vi "SIFT.vi"() -> ()   [LabVIEW 2018]
doc: "SIFT: This example is the SIFT feature detection example, which reads the image and converts it into a grayscale image, instantiates SIFT, detects key points, and draws the key point detection results on the image (only the middle point is drawn for each key point)"
uses:
  vi.lib/VIRobotics/opencv_yiku/ctls/KeyPoint.ctl
  vi.lib/VIRobotics/opencv_yiku/ctls/Point2f.ctl
  vi.lib/VIRobotics/opencv_yiku/ctls/ColorConversionCodes.ctl
  vi.lib/VIRobotics/opencv_yiku/Mat/Mat_8U/Mat_8U.lvclass
  C:/Program Files/National Instruments/LabVIEW 2018/vi.lib/VIRobotics/opencv_yiku/Mat/Mat/Mat.lvclass
  vi.lib/VIRobotics/opencv_yiku/Mat/Create_Mat_8U.vi
  vi.lib/VIRobotics/opencv_yiku/features2d/vector_KeyPoints/vector_KeyPoint_get_KeyPoints.vi
  vi.lib/VIRobotics/opencv_yiku/opencv_yiku.lvlib
  vi.lib/VIRobotics/opencv_yiku/features2d/SIFT/SIFT.lvclass
  vi.lib/VIRobotics/opencv_yiku/features2d/vector_KeyPoints/vector_KeyPoint.lvclass
panel:
  in  "nfeatures":i32=100
  out "src":picture
  out "SIFT_pic":picture
  out "KeyPoints1":T1[](array[typedef])
  # "Overview: Demonstrates how to find SIFT Keypoints and Descriptors\nRequirements: Windows.\nInstructions: \n1.Run the VI"
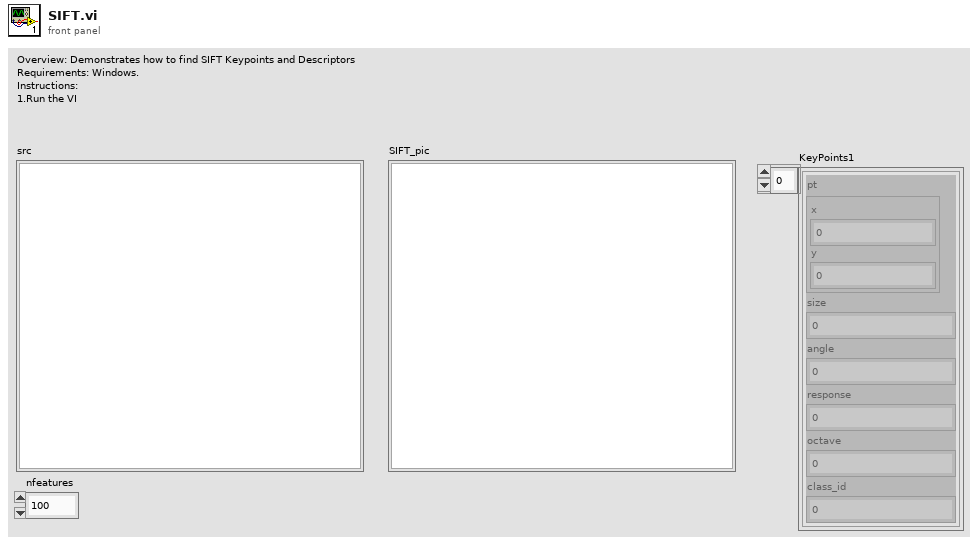
[diagram p1: front panel]
types:
  T1 = typedef "opencv_yiku.lvlib/KeyPoint.ctl" = cluster{"pt":T2, "size":sgl, "angle":sgl, "response":sgl, "octave":i32, "class_id":i32}
  T2 = typedef "opencv_yiku.lvlib/Point2f.ctl" = cluster{"x":sgl, "y":sgl}
  T3 = typedef "opencv_yiku.lvlib/ColorConversionCodes.ctl" = enum32{"COLOR_BGR2BGRA", "COLOR_BGRA2BGR", "COLOR_BGR2RGBA", "COLOR_RGBA2BGR", "COLOR_BGR2RGB", "COLOR_BGRA2RGBA", "COLOR_BGR2GRAY", "COLOR_RGB2GRAY", "COLOR_GRAY2BGR", "COLOR_GRAY2BGRA", "COLOR_BGRA2GRAY", "COLOR_RGBA2GRAY", "COLOR_BGR2BGR565", "COLOR_RGB2BGR565", "COLOR_BGR5652BGR", "COLOR_BGR5652RGB", "COLOR_BGRA2BGR565", "COLOR_RGBA2BGR565", "COLOR_BGR5652BGRA", "COLOR_BGR5652RGBA", "COLOR_GRAY2BGR565", "COLOR_BGR5652GRAY", "COLOR_BGR2BGR555", "COLOR_RGB2BGR555", "COLOR_BGR5552BGR", "COLOR_BGR5552RGB", "COLOR_BGRA2BGR555", "COLOR_RGBA2BGR555", "COLOR_BGR5552BGRA", "COLOR_BGR5552RGBA", "COLOR_GRAY2BGR555", "COLOR_BGR5552GRAY", "COLOR_BGR2XYZ", "COLOR_RGB2XYZ", "COLOR_XYZ2BGR", "COLOR_XYZ2RGB", "COLOR_BGR2YCrCb", "COLOR_RGB2YCrCb", "COLOR_YCrCb2BGR", "COLOR_YCrCb2RGB", "COLOR_BGR2HSV", "COLOR_RGB2HSV", "42", "43", "COLOR_BGR2Lab", "COLOR_RGB2Lab"}
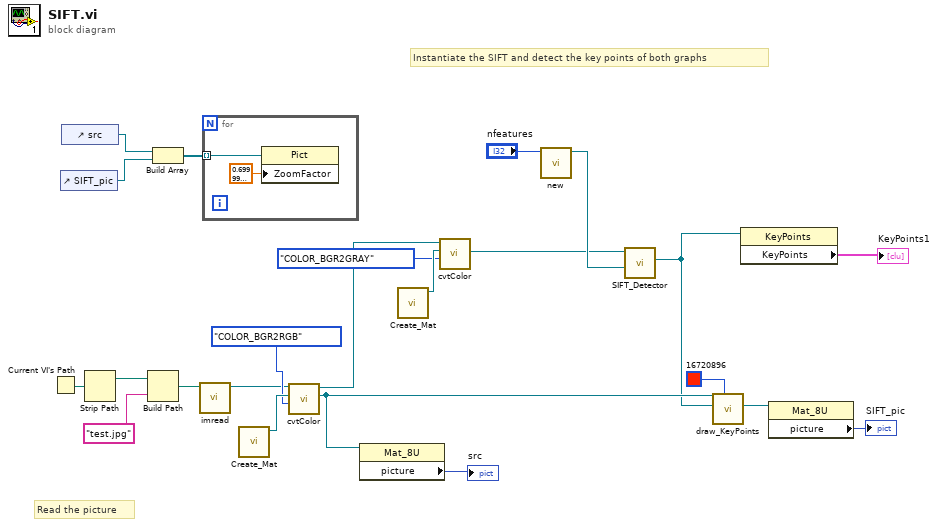
[diagram p0: block diagram]
diagram:
  # "Instantiate the SIFT and detect the key points of both graphs"
  # "Read the picture"
  n1 = Current VI's Path() -> (path=w20:path)
  n2 = control-ref of="SIFT_pic"() -> (w5:refnum<vi>)
  n3 = control-ref of="src"() -> (w6:refnum<vi>)
  n4 = Strip Path(path=w20) -> (stripped path=w17:path)  [unwired: 1 out]
  n5 = Build Path(base path=w17, name or relative path="test.jpg") -> (appended path=w18:path)
  n6 = Build Array(w6, w5) -> (w4:refnum<vi>[])
  n7 = call "imread.vi"("path"=w18) -> ("Mat out"=w10:refnum<class "Mat_8U.lvclass">)  [unwired: 9 in, 1 out]
  n8 = for {
    tunnel: w4 -> [w25] mode=indexing
    n9 = property class="Pict"(reference=w25, "ZoomFactor"=sgl 0.7 ("Zoom Factor")) -> ()  [unwired: 1 in, 2 out]
  }
  n10 = call-poly "Create_Mat.vi"() -> ("Mat_8U_out"=w12:refnum<class "Mat_8U.lvclass">)  [unwired: 10 in, 1 out]
  n11 = call "cvtColor.vi"("dstCn"=ColorConversionCodes."COLOR_BGR2RGB", "dst"=w12, "src"=w10) -> ("dst out"=w7:refnum<class "Mat_8U.lvclass">, "src out"=w8:refnum<class "Mat_8U.lvclass">)  [unwired: 6 in, 1 out]
  n12 = property class="Mat_8U"(reference=w7) -> ("picture"=→"src":picture)  [unwired: 1 in, 2 out]
  n13 = call-poly "Create_Mat.vi"() -> ("Mat_8U_out"=w15:refnum<class "Mat_8U.lvclass">)  [unwired: 10 in, 1 out]
  n14 = call "cvtColor.vi"("dstCn"=ColorConversionCodes."COLOR_BGR2GRAY", "dst"=w15, "src"=w8) -> ("dst out"=w13:refnum<class "Mat_8U.lvclass">)  [unwired: 6 in, 2 out]
  n15 = call "new.vi"("nfeatures"="nfeatures") -> ("SIFT out"=w23:refnum<class "SIFT.lvclass">)  [unwired: 9 in, 1 out]
  n16 = call "SIFT_Detector.vi"("SIFT"=w23, "img"=w13) -> ("vector_KeyPoint out"=w2:refnum<class "vector_KeyPoint.lvclass">)  [unwired: 6 in, 3 out]
  n17 = call "draw_KeyPoints.vi"("color"=u32 16720896, "vector_KeyPoint"=w2, "img"=w7) -> ("dst out"=w22:refnum<class "Mat_8U.lvclass">)  [unwired: 6 in, 2 out]
  n18 = property class="KeyPoints"(reference=w2) -> ("KeyPoints"=→"KeyPoints1":T1[])  [unwired: 1 in, 2 out]
  n19 = property class="Mat_8U"(reference=w22) -> ("picture"=→"SIFT_pic":picture)  [unwired: 1 in, 2 out]
